vi "DestroyClone.vi"(8 "error in (no error)":errorcluster, 9 "Exit via Stop Module Req?":bool, 10 "Wait for Module to stop?":bool, 11 "ModuleAdmin":refnum<class "ModuleAdmin.lvclass">) -> (0 "error out":errorcluster, 1 "External Launch":bool, 3 "Mod Admin out":refnum<class "ModuleAdmin.lvclass">)   [LabVIEW 2018, in "SensorPlugins.lvlib"]
uses:
  SensorPlugins.lvlib
  <userlib>/NIST/ModuleAdminLib/ModuleAdmin/ModuleAdmin.lvclass
  C:/Program Files (x86)/National Instruments/LabVIEW 2018/user.lib/NIST/ModuleAdminLib/ModuleAdminBase/ModuleAdminBase.lvclass
  <userlib>/NIST/ModuleAdminLib/ModuleAdmin/ModuleAdmin.lvclass/ModuleAdmin.ctl
  <userlib>/NIST/ModuleAdminLib/ModuleAdmin/Accessors/Read CloneRegRef.vi
  <userlib>/NIST/ModuleAdminLib/CloneRegistration/CloneRegistration.lvclass
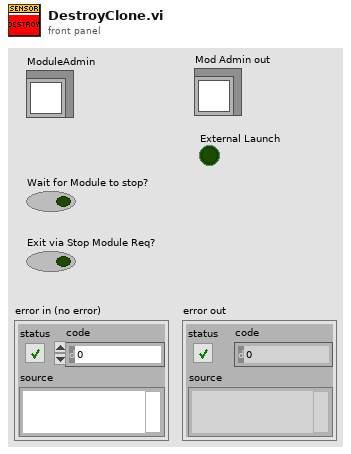
[diagram p1: front panel]
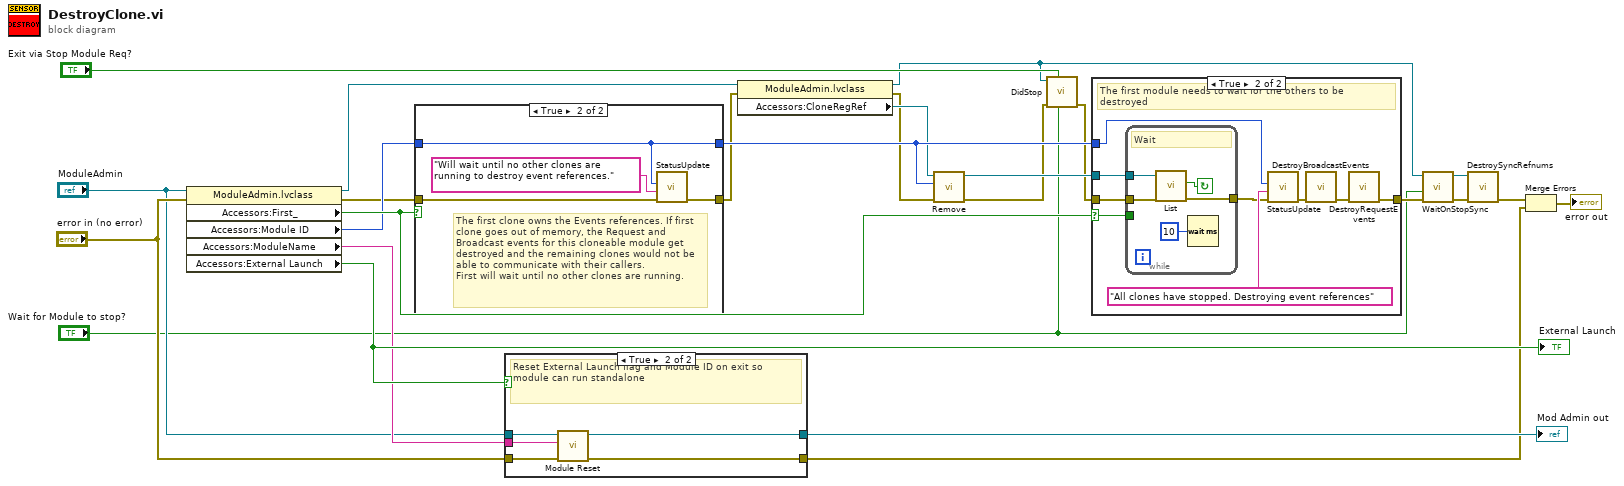
[diagram p0: block diagram]
diagram:
  n1 = property class="ModuleAdmin.lvclass"(reference="ModuleAdmin", error in="error in (no error)") -> (reference out=w6:refnum<class "ModuleAdmin.lvclass">, error out=w10:errorcluster, "Accessors:First_"=w25:bool, "Accessors:Module ID"=w16:i32, "Accessors:ModuleName"=w20:string, "Accessors:External Launch"=w22:bool)
  "External Launch" <- w22
  n2 = case shown="True" w25 {
    tunnel: w10 -> [w27 w31]
    tunnel: w16 -> [w26 w28]
    tunnel: [w27 w29] -> w5
    tunnel: [w26 w28] -> w24
    frame False {
    }
    frame True {
      # "The first clone owns the Events references. If first clone goes out of memory, the Request and Broadcast events for this cloneable module get destroyed and the remaining clones would not be able to communicate with their callers.\nFirst will wait until no other clones are running."
      n3 = call "StatusUpdate.vi"("error in (no error)"=w31, "Status"="Will wait until no other clones are running to destroy event references." ("format string"), "ModuleID"=w28) -> ("error out"=w29:errorcluster)  [unwired: 8 in]
    }
  }
  n4 = case shown="True" w22 {
    tunnel: "error in (no error)" -> [w32 w38]
    tunnel: w20 -> [_ w37]
    tunnel: "ModuleAdmin" -> [w33 w36]
    tunnel: [w33 w35] -> w19
    tunnel: [w32 w34] -> w17
    frame False {
    }
    frame True {
      # "Reset External Launch flag and Module ID on exit so module can run standalone"
      n5 = call <userlib>:"Module Reset.vi"("error in (no error)"=w38, "ModuleName"=w37, "Mod Admin in"=w36) -> ("error out"=w34:errorcluster, "Mod Admin out"=w35:refnum<class "ModuleAdmin.lvclass">)  [unwired: 7 in]
    }
  }
  "Mod Admin out" <- w19
  n6 = property class="ModuleAdmin.lvclass"(reference=w6, error in=w5) -> (reference out=w1:refnum<class "ModuleAdmin.lvclass">, error out=w4:errorcluster, "Accessors:CloneRegRef"=w9:refnum<data-value>)
  n7 = call <userlib>:"Remove.vi"("error in (no error)"=w4, "Module ID"=w24, "CloneRegRef"=w9) -> ("error out"=w13:errorcluster, "CloneRegRef"=w15:refnum<data-value>)  [unwired: 6 in, 1 out]
  n8 = call "DidStop.vi"("Wait for Module to stop?"="Wait for Module to stop?", "Exit via Stop Module Req?"="Exit via Stop Module Req?", "error in (no error)"=w13, "ModuleAdmin"=w1) -> ("error out"=w12:errorcluster)  [unwired: 7 in]
  n9 = case shown="True" w25 {
    selector: w25 -> [_ w47]
    tunnel: w12 -> [w39 w48]
    tunnel: w24 -> [_ w42]
    tunnel: [w39 w40] -> w8
    tunnel: w15 -> [_ w41]
    frame False {
    }
    frame True {
      # "The first module needs to wait for the others to be destroyed"
      n10 = while {
        tunnel: w48 -> [w53]
        tunnel: w47 -> [_]
        tunnel: [w52] -> w45
        tunnel: w41 -> [w49]
        stop <- w51 continue-if-true
        # "Wait"
        n11 = call <userlib>:"List.vi"("error in (no error)"=w53, "CloneRegRef"=w49) -> ("error out"=w52:errorcluster, "Found?"=w51:bool)  [unwired: 4 in, 4 out]
        n12 = Wait (ms)(milliseconds to wait=u32 10) -> ()  [unwired: 1 out]
      }
      n13 = call "StatusUpdate.vi"("error in (no error)"=w45, "Status"="All clones have stopped. Destroying event references", "ModuleID"=w42) -> ("error out"=w44:errorcluster)  [unwired: 8 in]
      n14 = call "DestroyBroadcastEvents.vi"("error in (no error)"=w44) -> ("error out"=w43:errorcluster)  [unwired: 10 in]
      n15 = call "DestroyRequestEvents.vi"("error in (no error)"=w43) -> ("error out"=w40:errorcluster)  [unwired: 10 in]
    }
  }
  n16 = call <userlib>:"WaitOnStopSync.vi"("error in (no error)"=w8, "WaitForModuleToStop?"="Wait for Module to stop?", "ModuleAdmin"=w1) -> ("error out"=w23:errorcluster, "ModuleAdmin"=w3:refnum<class "ModuleAdmin.lvclass">)  [unwired: 7 in]
  n17 = call <userlib>:"DestroySyncRefnums.vi"("error in (no error)"=w23, "ModuleAdmin"=w3) -> ("error out"=w7:errorcluster)  [unwired: 9 in]
  n18 = Merge Errors(w7, w17) -> (→"error out":errorcluster)
